vi "Construct.vi"(9 "Paramters":string, 10 "FINS CMD":T1, 11 "FINS Header":T2 {"SNA" max=127 format="%x"; "SA2" max=254 step=1 format="%x"; "SA1" format="%x"; "DA2" max=254 step=1 format="%x"; "DA1" format="%x"; "DNA" max=127 step=1 format="%x"}) -> (1 "msg":string)   [LabVIEW 2020, in "FINS TCP.lvlib"]
uses:
  FINS TCP.lvlib
  FINS_header.ctl
  FINS CMD.ctl
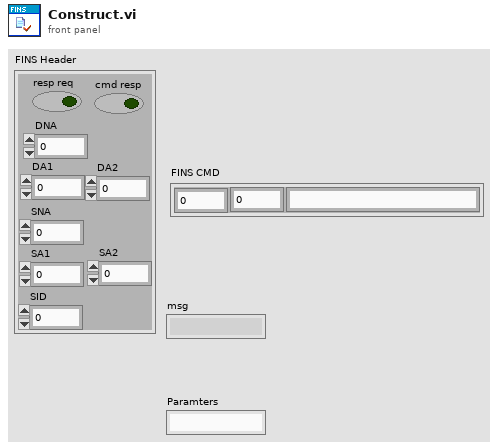
[diagram p1: front panel]
types:
  T1 = typedef "FINS TCP.lvlib/FINS CMD.ctl" = cluster{"MR":u8, "SR":u8, "name":string}
  T2 = typedef "FINS TCP.lvlib/FINS_header.ctl" = cluster{"resp req":bool, "cmd resp":bool, "SID":u8, "DNA":u8, "DA1":u8, "DA2":u8, "SA1":u8, "SA2":u8, "SNA":u8}
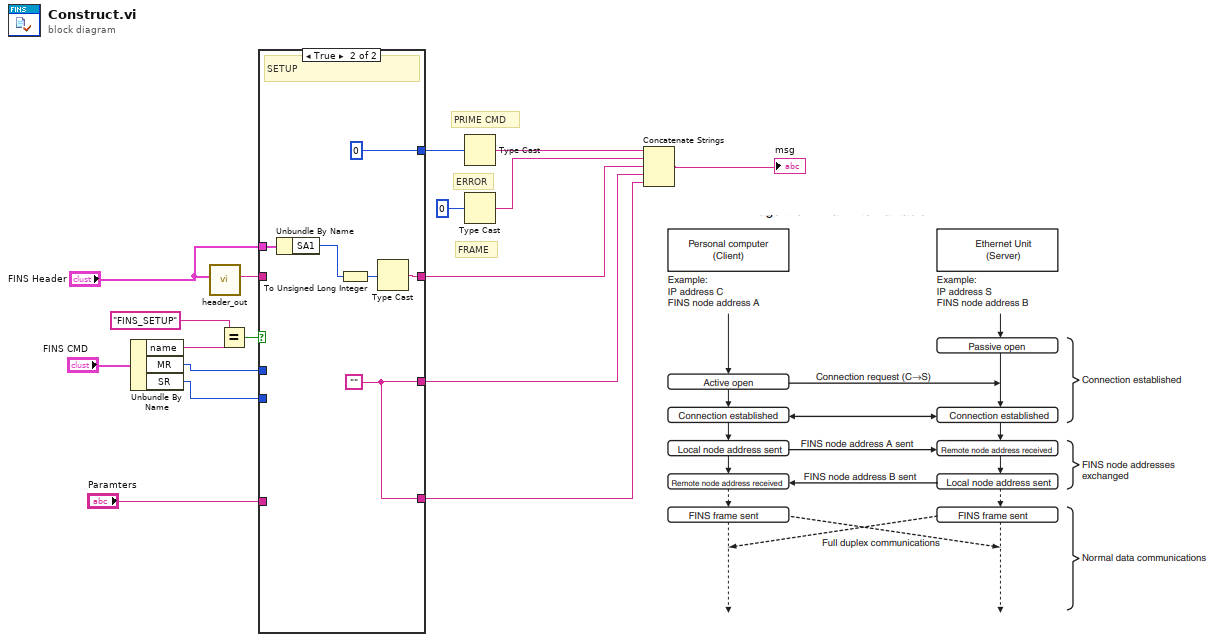
[diagram p0: block diagram]
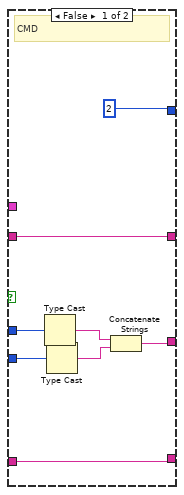
[diagram p2: hidden frame]
diagram:
  # "FRAME"
  # "PRIME CMD"
  # "ERROR"
  n1 = Unbundle By Name("FINS CMD") -> ("name"=w6:string, "MR"=w5:u8, "SR"=w4:u8)
  n2 = call "header_out.vi"("FINS Header"="FINS Header") -> ("FINS Header"=w17:string)  [unwired: 10 in]
  n3 = Equal?(x="FINS_SETUP", y=w6) -> (x = y?=w9:bool)
  n4 = case shown="True" w9 {
    tunnel: w17 -> [w25 _]
    tunnel: [w25 w30] -> w11
    tunnel: "FINS Header" -> [_ w31]
    tunnel: [u32 2 ("CMD") u32 0 ("CMD")] -> w14
    tunnel: "Paramters" -> [w23 _]
    tunnel: [w23 w28] -> w10
    tunnel: [w18 w28] -> w3
    tunnel: w5 -> [w20 _]
    tunnel: w4 -> [w19 _]
    frame False {
      # "CMD"
      n5 = Type Cast(x=w20) -> (*(type *) &x=w22:string)  [unwired: 1 in]
      n6 = Type Cast(x=w19) -> (*(type *) &x=w21:string)  [unwired: 1 in]
      n7 = Concatenate Strings(w22, w21) -> (w18:string)
    }
    frame True {
      w28 = ""
      # "SETUP"
      n8 = Unbundle By Name(w31) -> ("SA1"=w27:u8)
      n9 = To Unsigned Long Integer(number=w27) -> (unsigned 32bit integer=w26:u32)
      n10 = Type Cast(x=w26) -> (*(type *) &x=w30:string)  [unwired: 1 in]
    }
  }
  n11 = Type Cast(x=w14) -> (*(type *) &x=w13:string)  [unwired: 1 in]
  n12 = Type Cast(x=u32 0 ("length")) -> (*(type *) &x=w15:string)  [unwired: 1 in]
  n13 = Concatenate Strings(w13, w15, w11, w3, w10) -> (→"msg":string)
